vi "Facade.vi"(0 "Data In":T4 caption="数据输入", 2 "Display State In":T2 caption="显示状态输入", 3 "Container State":T3 caption="容器状态") -> (6 "Data Out":T4 caption="数据输出", 7 "Display State Out":T2 caption="显示状态输出", 8 "Action":T1={"Data Changed?"=TRUE, "State Changed?"=TRUE, "Action Name"=""} caption="动作")   [LabVIEW 2016, in "FalseColorEditer.xctl"]
uses:
  FalseColorEditer.xctl
  Data.ctl
  <vilib>/_xctls/Container State.ctl
  State.ctl
  <vilib>/_xctls/Action.ctl
  <vilib>/picture/picture.llb/Draw True-Color Pixmap.vi
  <vilib>/_xctls/XControlSupport.lvlib
panel:
  in  "Style":u16(ring)
  out "渐变图":picture
  out "曲线图":picture
  out "坐标":picture
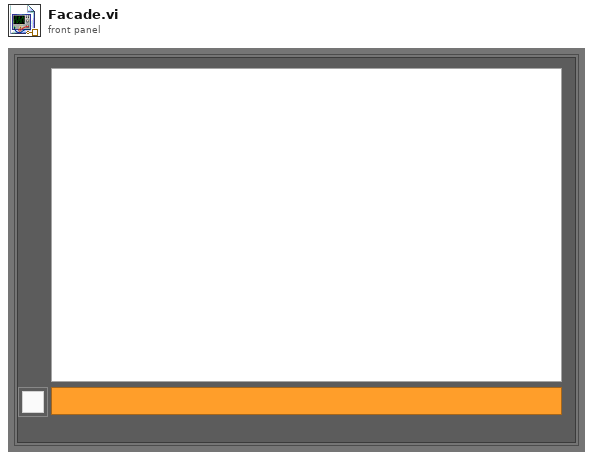
[diagram p1: front panel]
types:
  T1 = typedef "XControlSupport.lvlib/Action.ctl" = cluster{"Data Changed?":bool, "State Changed?":bool, "Action Name":string}
  T2 = typedef "FalseColorEditer.xctl/State.ctl" = cluster{"MousesPressDown?":bool, "ActiveCurveID":i8, "R Curve ":cluster{i16, i16}[], "G Curve":cluster{i16, i16}[], "B Curve":cluster{i16, i16}[]}
  T3 = typedef "XControlSupport.lvlib/Container State.ctl" = cluster{"Indicator?":bool, "Run Mode?":bool, " Refnum":refnum<vi>}
  T4 = typedef "FalseColorEditer.xctl/Data.ctl" = cluster{"Ratio_R":cluster{dbl, dbl}[], "Ratio_G":cluster{dbl, dbl}[], "Ratio_B":cluster{dbl, dbl}[]}
  T5 = cluster{"horizontal":bool, "left/top":bool, "draw bar":bool, "line color":u32, "text color(black)":u32}
  T6 = cluster{"coordinate 1":i16, "value 1":dbl, "coordinate 2":i16, "value 2":dbl, "log?(F)":bool, "fmt and prec":cluster{"format":enum8{"Decimal", "Scientific", "Engineering", "Binary", "Octal", "Hex"}, "precision":u8}}
  T7 = typedef "LVBoundsTypeDef.ctl" = cluster{"Width":u32, "Height":u32}
  T8 = cluster{cluster{dbl, "R":dbl}[], cluster{dbl, "G":dbl}[], cluster{dbl, "B":dbl}[]}
  T9 = typedef "LVMouseTypeDef.ctl" = cluster{"Mouse Position":cluster{"X":i32, "Y":i32}, "Mouse Modifiers":cluster{"Button Down":bool, "Shift Mod":bool, "Menu Mod":bool, "Option Mod":bool}}
  T10 = cluster{"RFalseColorRatioData":cluster{dbl, dbl}[], "GFalseColorRatioData":cluster{dbl, dbl}[], "BFalseColorRatioData":cluster{dbl, dbl}[]}
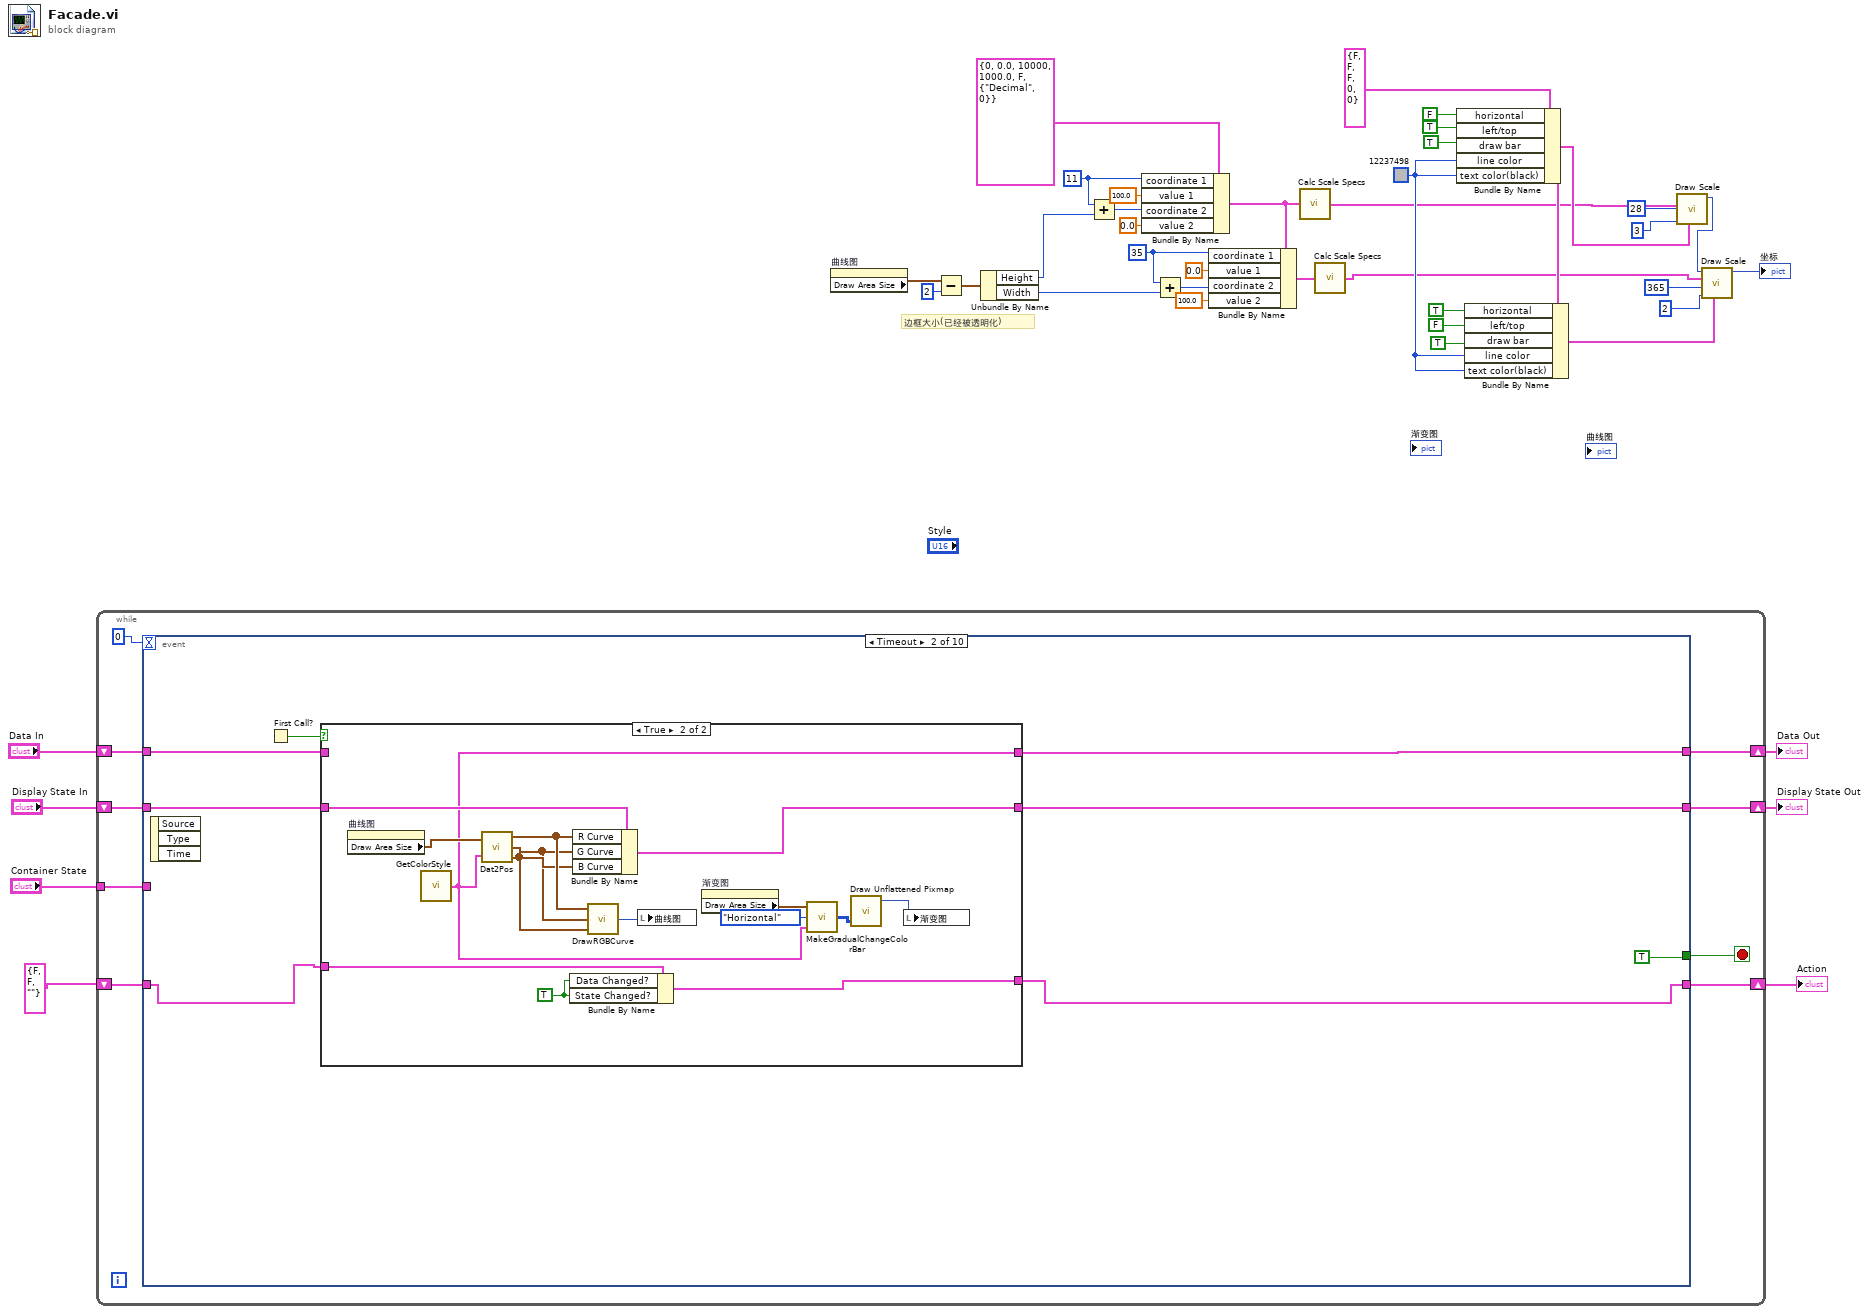
[diagram p0: block diagram]
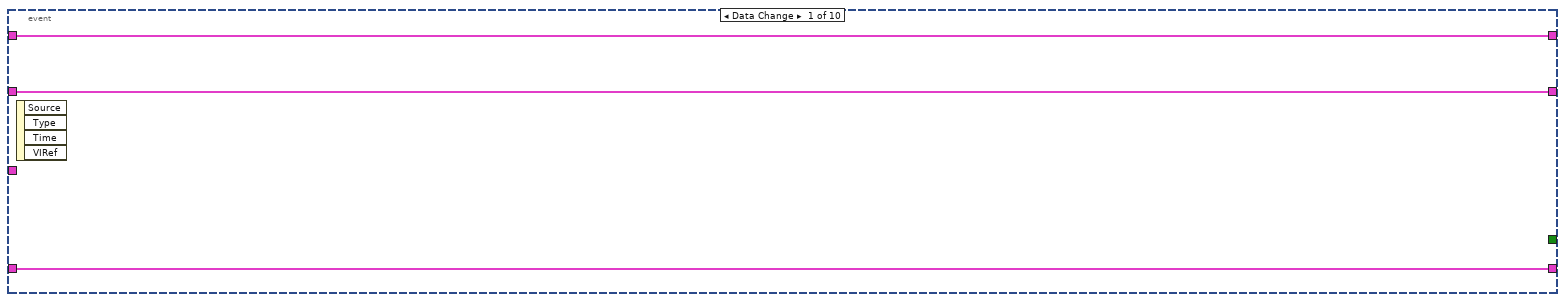
[diagram p2: hidden frame]
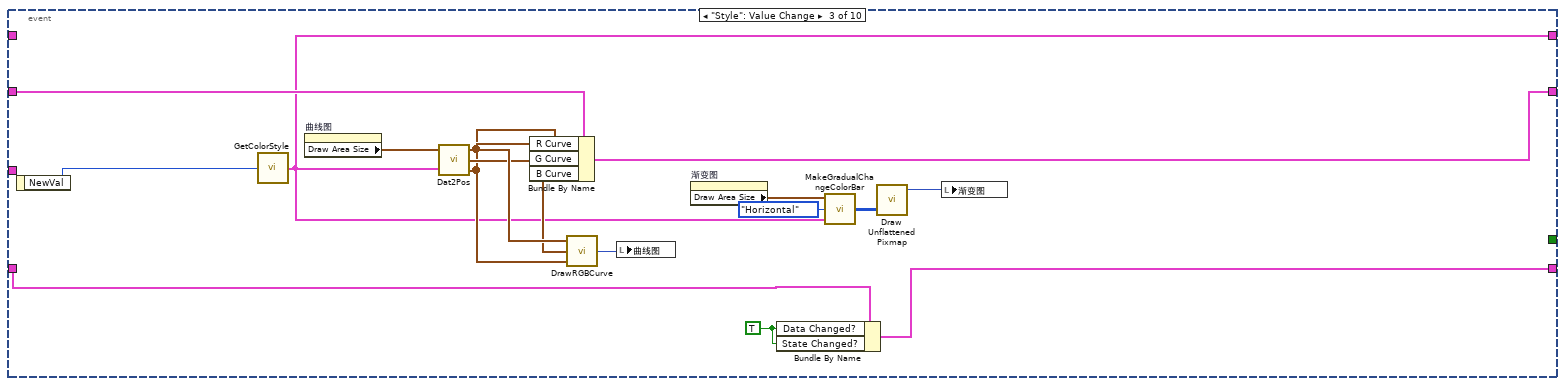
[diagram p4: hidden frame]
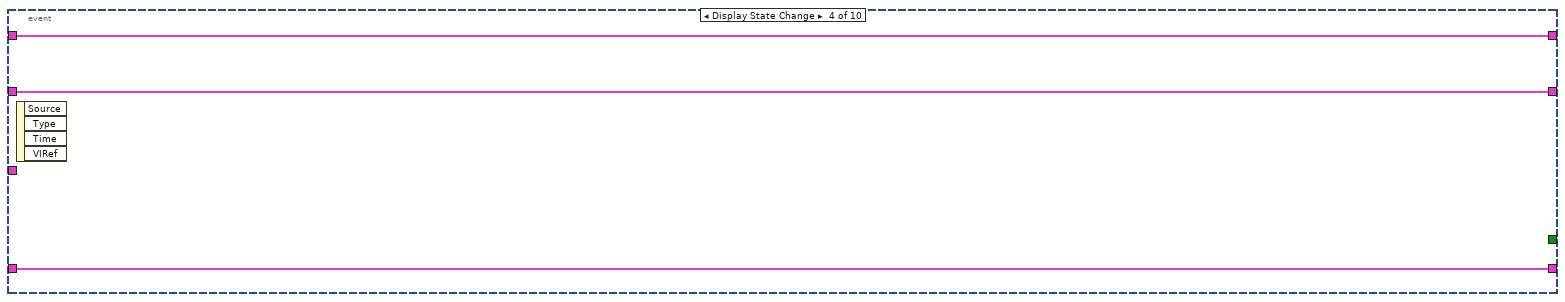
[diagram p5: hidden frame]
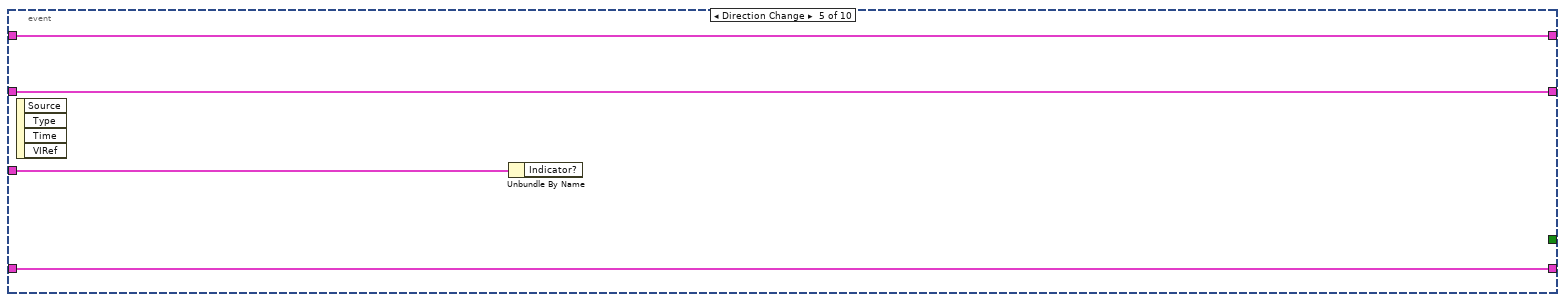
[diagram p6: hidden frame]
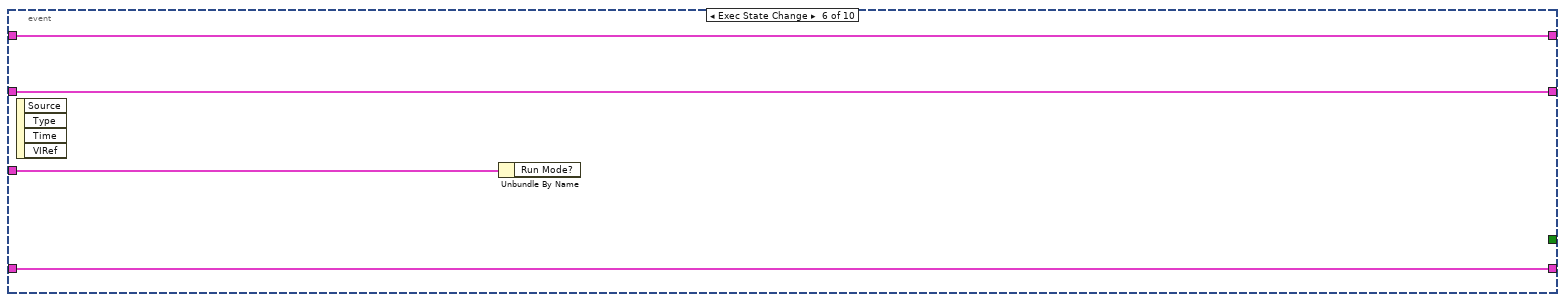
[diagram p7: hidden frame]
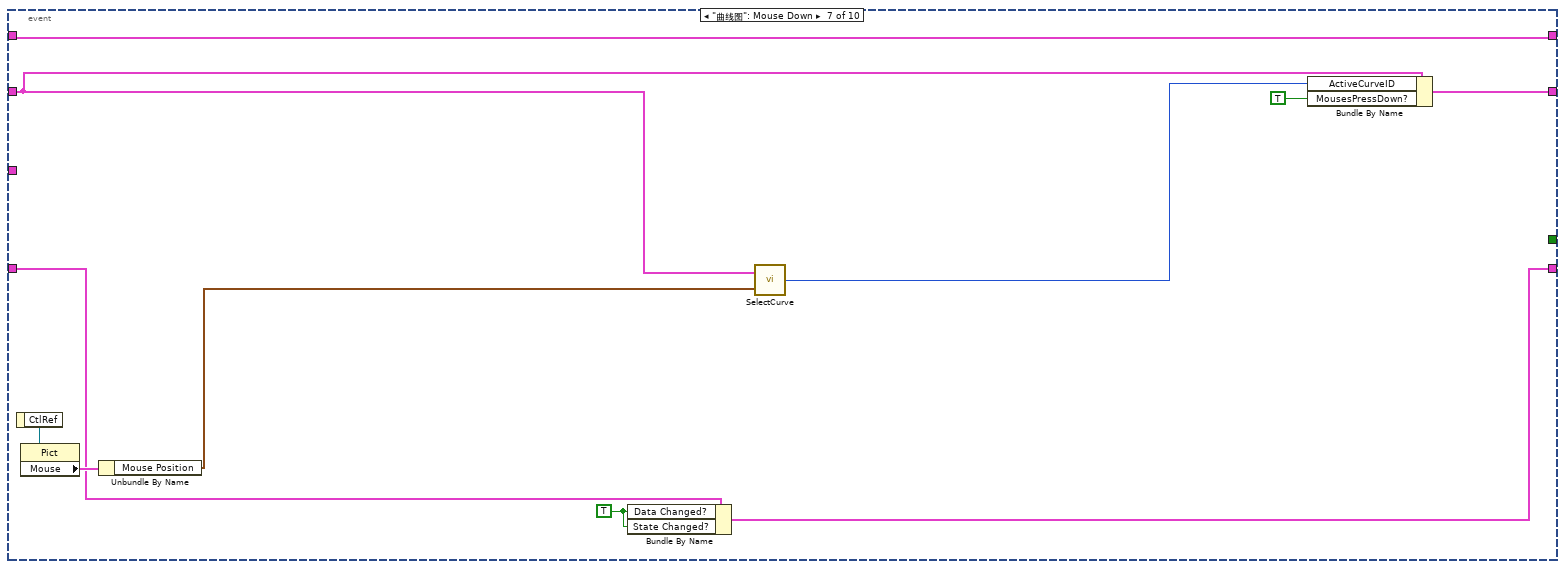
[diagram p8: hidden frame]
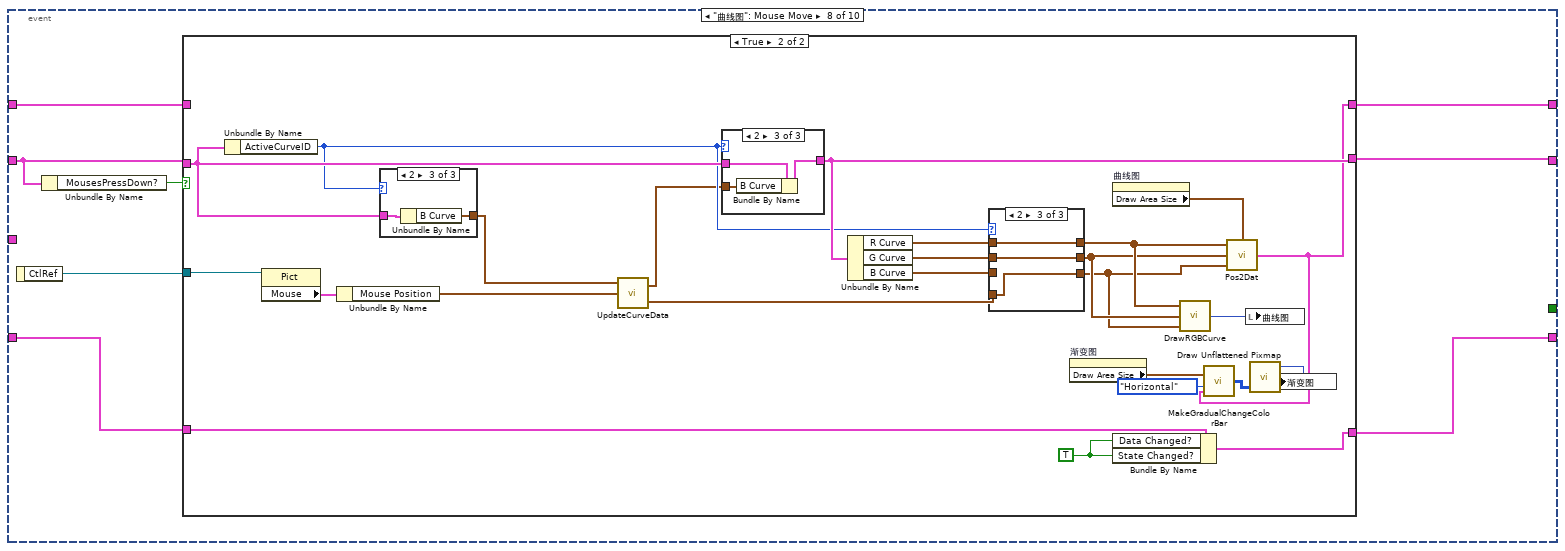
[diagram p9: hidden frame]
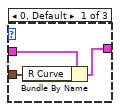
[diagram p13: hidden frame]
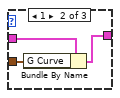
[diagram p14: hidden frame]
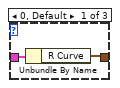
[diagram p15: hidden frame]
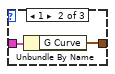
[diagram p16: hidden frame]
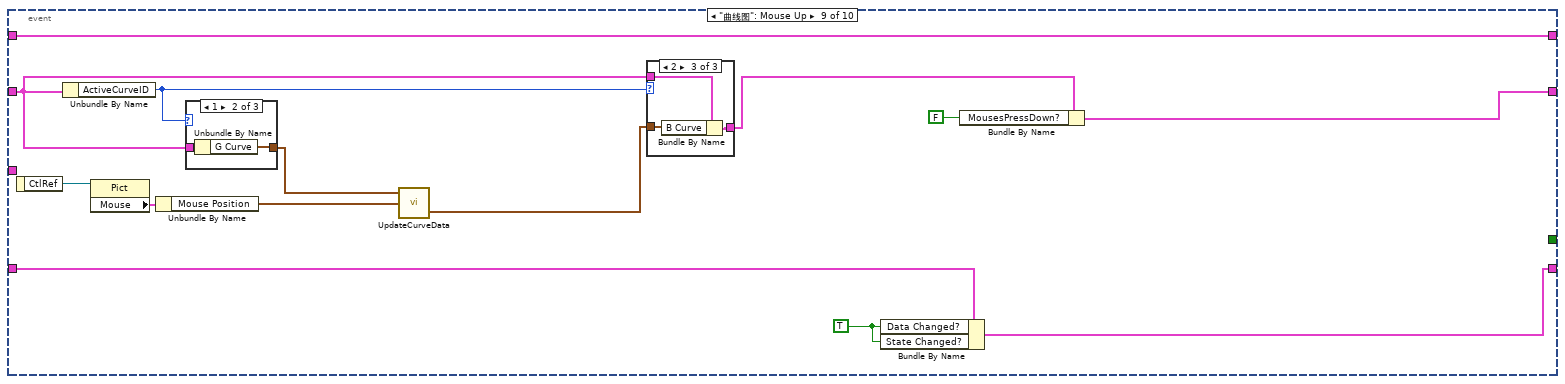
[diagram p17: hidden frame]
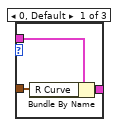
[diagram p18: hidden frame]
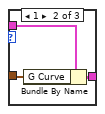
[diagram p19: hidden frame]
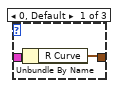
[diagram p20: hidden frame]
diagram:
  w29 = i16 11 ("precision")
  w25 = i16 35 ("precision")
  w9 = u32 12237498 ("line color")
  # "边框大小(已经被透明化)"
  n1 = while {
    shift-right: [w49] -> w38
    shift-left: "Display State In" -> [w50]
    tunnel: "Container State" -> [w46]
    shift-right: [w43] -> w41
    shift-left: "Data In" -> [w45]
    shift-right: [w42] -> w37
    shift-left: T1 {"Data Changed?"=FALSE, "State Changed?"=FALSE, "Action Name"=""} ("Action") -> [w44]
    stop <- w48 stop-if-true
    n2 = event shown="[1] Timeout" {
      selector: _ -> [_ _ _ _ _ _ _ _ _ _]
      dyn-events: _ -> [_ _ _ _ _ _ _ _ _ _]
      timeout: 0 -> [_ _ _ _ _ _ _ _ _ _]
      tunnel: w50 -> [w52 w59 w89 w98 w101 w105 w114 w120 w185 w208]
      tunnel: [w52 w58 w88 w98 w101 w105 w113 w124 w184 w207] -> w49
      tunnel: [_ TRUE _ _ _ _ _ _ _ _] -> w48
      tunnel: w46 -> [_ _ _ _ w102 w106 _ _ _ _]
      tunnel: w45 -> [w53 w57 _ w97 w100 w104 w117 w118 w181 w210]
      tunnel: [w53 w56 w87 w97 w100 w104 w117 w119 w181 w210] -> w43
      tunnel: w44 -> [w51 w55 w84 w96 w99 w103 w109 w123 w188 _]
      tunnel: [w51 w54 w83 w96 w99 w103 w108 w122 w189 _] -> w42
      event Data Change {
        n3 = event-data() -> ()  [unwired: 5 out]
      }
      event Timeout {
        n4 = event-data() -> ()  [unwired: 4 out]
        n5 = First Call?() -> (First Call?: T/F=w60:bool)
        n6 = case shown="True" w60 {
          tunnel: w59 -> [w64 w74]
          tunnel: [w64 w73] -> w58
          tunnel: w57 -> [w63 _]
          tunnel: [w63 w72] -> w56
          tunnel: w55 -> [w62 w67]
          tunnel: [w62 w66] -> w54
          frame False {
          }
          frame True {
            w65 = TRUE ("State Changed?")
            n7 = property on="曲线图" class="Pict"() -> ("Draw Area Size"=w79:T7)  [unwired: 2 in, 2 out]
            n8 = call "GetColorStyle.vi"() -> ("FalseColorData"=w72:T8)  [unwired: 1 in]
            n9 = call "Dat2Pos.vi"("Draw Area Size"=w79, "FalseColorRatioData"=w72) -> ("R MappedPostionInPicture"=w78:cluster{i16, i16}[], "G MappedPostionInPicture"=w71:cluster{i16, i16}[], "B MappedPostionInPicture"=w77:cluster{i16, i16}[])
            n10 = Bundle By Name(cluster=w67, "Data Changed?"=w65, "State Changed?"=w65) -> (w66:T1)
            n11 = Bundle By Name(cluster=w74, "R Curve"=w78, "G Curve"=w71, "B Curve"=w77) -> (w73:T2)
            n12 = call "DrawRGBCurve.vi"("BCurvePos"=w77, "GCurvePos"=w71, "RCurvePos"=w78) -> ("Curve in picture"=w76:picture)
            n13 = local write "曲线图"(w76) -> ()
            n14 = property on="渐变图" class="Pict"() -> ("Draw Area Size"=w75:T7)  [unwired: 2 in, 2 out]
            n15 = call "MakeGradualChangeColorBar.vi"("FalseColorData"=w72, "Direction"=enum16{"Horizontal", "Vertical"}."Horizontal", "GradualChangeColorBar Size"=w75) -> ("GradualChangeColorBarPicDat"=w69:u32[][])
            n16 = call-poly <vilib>:"Draw Unflattened Pixmap.vi"("data (RGB format)"=w69) -> ("new picture"=w68:picture)  [unwired: 3 in, 5 out]
            n17 = local write "渐变图"(w68) -> ()
          }
        }
      }
      event "Style": Value Change {
        w86 = TRUE ("Data Changed?")
        n18 = event-data() -> ("NewVal"=w85:u16)  [unwired: 1 out]
        n19 = call "GetColorStyle.vi"("ColorStyle"=w85) -> ("FalseColorData"=w87:T8)
        n20 = property on="曲线图" class="Pict"() -> ("Draw Area Size"=w95:T7)  [unwired: 2 in, 2 out]
        n21 = call "Dat2Pos.vi"("Draw Area Size"=w95, "FalseColorRatioData"=w87) -> ("R MappedPostionInPicture"=w94:cluster{i16, i16}[], "G MappedPostionInPicture"=w93:cluster{i16, i16}[], "B MappedPostionInPicture"=w92:cluster{i16, i16}[])
        n22 = Bundle By Name(cluster=w89, "R Curve"=w94, "G Curve"=w93, "B Curve"=w92) -> (w88:T2)
        n23 = call "DrawRGBCurve.vi"("BCurvePos"=w92, "GCurvePos"=w93, "RCurvePos"=w94) -> ("Curve in picture"=w91:picture)
        n24 = local write "曲线图"(w91) -> ()
        n25 = property on="渐变图" class="Pict"() -> ("Draw Area Size"=w90:T7)  [unwired: 2 in, 2 out]
        n26 = Bundle By Name(cluster=w84, "Data Changed?"=w86, "State Changed?"=w86) -> (w83:T1)
        n27 = call "MakeGradualChangeColorBar.vi"("FalseColorData"=w87, "Direction"=enum16{"Horizontal", "Vertical"}."Horizontal", "GradualChangeColorBar Size"=w90) -> ("GradualChangeColorBarPicDat"=w81:u32[][])
        n28 = call-poly <vilib>:"Draw Unflattened Pixmap.vi"("data (RGB format)"=w81) -> ("new picture"=w80:picture)  [unwired: 3 in, 5 out]
        n29 = local write "渐变图"(w80) -> ()
      }
      event Display State Change {
        n30 = event-data() -> ()  [unwired: 5 out]
      }
      event Direction Change {
        n31 = event-data() -> ()  [unwired: 5 out]
        n32 = Unbundle By Name(w102) -> ()  [unwired: 1 out]
      }
      event Exec State Change {
        n33 = event-data() -> ()  [unwired: 5 out]
        n34 = Unbundle By Name(w106) -> ()  [unwired: 1 out]
      }
      event "曲线图": Mouse Down {
        w107 = TRUE ("Data Changed?")
        n35 = event-data() -> ("CtlRef"=w110:refnum<vi>)  [unwired: 1 out]
        n36 = property class="Pict"(reference=w110) -> ("Mouse"=w116:T9)  [unwired: 1 in, 2 out]
        n37 = Unbundle By Name(w116) -> ("Mouse Position"=w115:cluster{"X":i32, "Y":i32})
        n38 = Bundle By Name(cluster=w109, "Data Changed?"=w107, "State Changed?"=w107) -> (w108:T1)
        n39 = call "SelectCurve.vi"("Mouse Position"=w115, "Display State In"=w114) -> ("MinDistanceID"=w112:u8)
        n40 = Bundle By Name(cluster=w114, "ActiveCurveID"=w112, "MousesPressDown?"=TRUE ("MouseHasPressDown?")) -> (w113:T2)
      }
      event "曲线图": Mouse Move {
        n41 = event-data() -> ("CtlRef"=w125:refnum<vi>)  [unwired: 1 out]
        n42 = Unbundle By Name(w120) -> ("MousesPressDown?"=w121:bool)
        n43 = case shown="True" w121 {
          tunnel: w125 -> [_ w142]
          tunnel: w120 -> [w128 w148]
          tunnel: [w128 w147] -> w124
          tunnel: w123 -> [w127 w152]
          tunnel: [w127 w151] -> w122
          tunnel: w118 -> [w126 _]
          tunnel: [w126 w135] -> w119
          frame False {
          }
          frame True {
            w150 = TRUE ("Data Changed?")
            n44 = Unbundle By Name(w148) -> ("ActiveCurveID"=w146:i8)
            n45 = property class="Pict"(reference=w142) -> ("Mouse"=w153:T9)  [unwired: 1 in, 2 out]
            n46 = Unbundle By Name(w153) -> ("Mouse Position"=w140:cluster{"X":i32, "Y":i32})
            n47 = case shown="2" w146 {
              tunnel: w148 -> [w173 w175 w177]
              tunnel: [w172 w174 w176] -> w141
              frame 0, Default {
                n48 = Unbundle By Name(w173) -> ("R Curve"=w172:cluster{i16, i16}[])
              }
              frame 1 {
                n49 = Unbundle By Name(w175) -> ("G Curve"=w174:cluster{i16, i16}[])
              }
              frame 2 {
                n50 = Unbundle By Name(w177) -> ("B Curve"=w176:cluster{i16, i16}[])
              }
            }
            n51 = call "UpdateCurveData.vi"("Mouse Position"=w140, "Curve Data"=w141) -> ("Refresh Curve Data"=w134:cluster{i16, i16}[], "Curve Data Out"=w133:cluster{i16, i16}[])  [unwired: 1 in]
            n52 = case shown="2" w146 {
              tunnel: w148 -> [w165 w168 w171]
              tunnel: [w164 w167 w170] -> w147
              tunnel: w133 -> [w163 w166 w169]
              frame 0, Default {
                n53 = Bundle By Name(cluster=w165, "R Curve"=w163) -> (w164:T2)
              }
              frame 1 {
                n54 = Bundle By Name(cluster=w168, "G Curve"=w166) -> (w167:T2)
              }
              frame 2 {
                n55 = Bundle By Name(cluster=w171, "B Curve"=w169) -> (w170:T2)
              }
            }
            n56 = Unbundle By Name(w147) -> ("R Curve"=w145:cluster{i16, i16}[], "G Curve"=w144:cluster{i16, i16}[], "B Curve"=w143:cluster{i16, i16}[])
            n57 = case shown="2" w146 {
              tunnel: w145 -> [_ w159 w160]
              tunnel: w144 -> [w155 _ w161]
              tunnel: w143 -> [w154 w158 _]
              tunnel: w134 -> [w156 w157 w162]
              tunnel: [w156 w159 w160] -> w139
              tunnel: [w155 w157 w161] -> w138
              tunnel: [w154 w158 w162] -> w137
              frame 0, Default {
              }
              frame 1 {
              }
              frame 2 {
              }
            }
            n58 = property on="渐变图" class="Pict"() -> ("Draw Area Size"=w132:T7)  [unwired: 2 in, 2 out]
            n59 = property on="曲线图" class="Pict"() -> ("Draw Area Size"=w136:T7)  [unwired: 2 in, 2 out]
            n60 = Bundle By Name(cluster=w152, "Data Changed?"=w150, "State Changed?"=w150) -> (w151:T1)
            n61 = call "DrawRGBCurve.vi"("BCurvePos"=w137, "GCurvePos"=w138, "RCurvePos"=w139) -> ("Curve in picture"=w149:picture)
            n62 = call "Pos2Dat.vi"("Draw Area Size"=w136, "BCurvePosInPic"=w137, "GCurvePosInPic"=w138, "RCurvePosInPic"=w139) -> ("FalseColorRatioData"=w135:T10)
            n63 = call "MakeGradualChangeColorBar.vi"("FalseColorData"=w135, "Direction"=enum16{"Horizontal", "Vertical"}."Horizontal", "GradualChangeColorBar Size"=w132) -> ("GradualChangeColorBarPicDat"=w130:u32[][])
            n64 = local write "曲线图"(w149) -> ()
            n65 = call-poly <vilib>:"Draw Unflattened Pixmap.vi"("data (RGB format)"=w130) -> ("new picture"=w129:picture)  [unwired: 3 in, 5 out]
            n66 = local write "渐变图"(w129) -> ()
          }
        }
      }
      event "曲线图": Mouse Up {
        w187 = TRUE ("Data Changed?")
        n67 = event-data() -> ("CtlRef"=w190:refnum<vi>)  [unwired: 1 out]
        n68 = Unbundle By Name(w185) -> ("ActiveCurveID"=w186:i8)
        n69 = property class="Pict"(reference=w190) -> ("Mouse"=w191:T9)  [unwired: 1 in, 2 out]
        n70 = Unbundle By Name(w191) -> ("Mouse Position"=w179:cluster{"X":i32, "Y":i32})
        n71 = case shown="1" w186 {
          tunnel: w185 -> [w202 w204 w206]
          tunnel: [w201 w203 w205] -> w180
          frame 0, Default {
            n72 = Unbundle By Name(w202) -> ("R Curve"=w201:cluster{i16, i16}[])
          }
          frame 1 {
            n73 = Unbundle By Name(w204) -> ("G Curve"=w203:cluster{i16, i16}[])
          }
          frame 2 {
            n74 = Unbundle By Name(w206) -> ("B Curve"=w205:cluster{i16, i16}[])
          }
        }
        n75 = call "UpdateCurveData.vi"("Mouse Position"=w179, "Curve Data"=w180) -> ("Refresh Curve Data"=w178:cluster{i16, i16}[])  [unwired: 1 in, 1 out]
        n76 = case shown="2" w186 {
          tunnel: [w194 w197 w200] -> w182
          tunnel: w185 -> [w193 w196 w199]
          tunnel: w178 -> [w192 w195 w198]
          frame 0, Default {
            n77 = Bundle By Name(cluster=w193, "R Curve"=w192) -> (w194:T2)
          }
          frame 1 {
            n78 = Bundle By Name(cluster=w196, "G Curve"=w195) -> (w197:T2)
          }
          frame 2 {
            n79 = Bundle By Name(cluster=w199, "B Curve"=w198) -> (w200:T2)
          }
        }
        n80 = Bundle By Name(cluster=w188, "Data Changed?"=w187, "State Changed?"=w187) -> (w189:T1)
        n81 = Bundle By Name(cluster=w182, "MousesPressDown?"=FALSE) -> (w184:T2)
      }
      event "曲线图": Mouse Leave {
        n82 = event-data() -> ()  [unwired: 5 out]
        n83 = Bundle By Name(cluster=w208, "MousesPressDown?"=FALSE) -> (w207:T2)
      }
    }
  }
  "Display State Out" <- w38
  "Data Out" <- w41
  "Action" <- w37
  n84 = property on="曲线图" class="Pict"() -> ("Draw Area Size"=w19:T7)  [unwired: 2 in, 2 out]
  n85 = Subtract(x=w19, y=u32 2) -> (x-y=w18:T7)
  n86 = Unbundle By Name(w18) -> ("Height"=w17:u32, "Width"=w16:u32)
  n87 = Add(x=w29, y=w17) -> (x+y=w8:u32)
  n88 = Bundle By Name(cluster=T6 {"coordinate 1"=0, "value 1"=0.0, "coordinate 2"=10000, "value 2"=1000.0, "log?(F)"=FALSE, "fmt and prec"={"format"=enum."Decimal", "precision"=0}} ("scale definition"), "coordinate 1"=w29, "value 1"=100.0 ("precision"), "coordinate 2"=w8, "value 2"=0.0 ("precision")) -> (w22:T6)
  n89 = Add(x=w25, y=w16) -> (x+y=w24:u32)
  n90 = Bundle By Name(cluster=w22, "coordinate 1"=w25, "value 1"=0.0 ("precision"), "coordinate 2"=w24, "value 2"=100.0 ("precision")) -> (w21:T6)
  n91 = call <vilib>:"Calc Scale Specs.vi"("scale definition"=w22) -> ("scale specs"=w5:cluster{"coordinate":i16, "label":string}[])  [unwired: 3 in, 5 out]
  n92 = call <vilib>:"Calc Scale Specs.vi"("scale definition"=w21) -> ("scale specs"=w4:cluster{"coordinate":i16, "label":string}[])  [unwired: 3 in, 5 out]
  n93 = Bundle By Name(cluster=T5 {"horizontal"=FALSE, "left/top"=FALSE, "draw bar"=FALSE, "line color"=0, "text color(black)"=0} ("scale attributes"), "horizontal"=FALSE, "left/top"=TRUE ("horizontal"), "draw bar"=TRUE ("horizontal"), "line color"=w9, "text color(black)"=w9) -> (w6:T5)
  n94 = Bundle By Name(cluster=w6, "horizontal"=TRUE, "left/top"=FALSE ("horizontal"), "draw bar"=TRUE ("horizontal"), "line color"=w9, "text color(black)"=w9) -> (w1:T5)
  n95 = call <vilib>:"Draw Scale.vi"("scale attributes"=w6, "tick length(3)"=i16 3, "constant coordinate"=i16 28, "scale specs"=w5) -> ("new picture"=w3:picture)  [unwired: 3 in, 4 out]
  n96 = call <vilib>:"Draw Scale.vi"("scale attributes"=w1, "tick length(3)"=i16 2, "constant coordinate"=i16 365, "scale specs"=w4, "picture"=w3) -> ("new picture"=→"坐标":picture)  [unwired: 2 in, 4 out]
